vi "Read from File.vi"(8 "error in (no error)":errorcluster, 10 "INI Ref":T1, 11 "Wait Action in":refnum<class "Wait Action.lvclass">) -> (0 "error out":errorcluster, 2 "INI Ref out":T1, 3 "Wait Action out":refnum<class "Wait Action.lvclass">)   [LabVIEW 2020, in "MacroAssert.lvlib" / "Wait Action.lvclass"]
uses:
  Wait Action.lvclass
  Wait Action.lvclass/Wait Action.ctl
  Macro Step/Macro Step.lvclass
  <vilib>/Utility/config.llb/Config Data RefNum.ctl
  <vilib>/Utility/config.llb/NI_LVConfig.lvlib
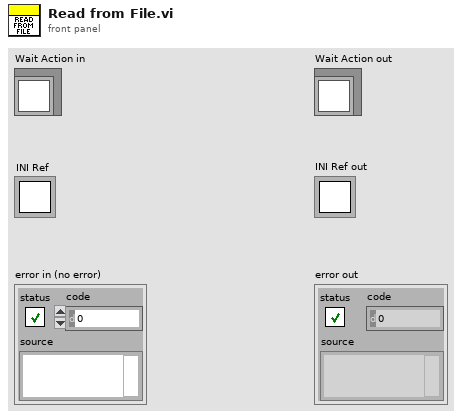
[diagram p1: front panel]
types:
  T1 = typedef "NI_LVConfig.lvlib/Config Data RefNum.ctl" = refnum<k1>
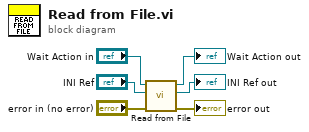
[diagram p0: block diagram]
diagram:
  n1 = call-parent "Read from File.vi"("error in (no error)"="error in (no error)", "INI Ref"="INI Ref", "Macro Step in"="Wait Action in") -> ("error out"=→"error out":errorcluster, "INI Ref out"=→"INI Ref out":T1, "Macro Step out"=→"Wait Action out":refnum<class "Wait Action.lvclass">)  [unwired: 6 in]
